vi "GetOneErrorData.vi"(8 "ErrorIn":errorcluster caption="Error In(no Error)", 9 "ErrorCode":i32, 11 "ReferenceIn":refnum<class "ErrorDefinitionSQLite.lvclass"> caption="Reference In") -> (0 "ErrorOut":errorcluster caption="Error Out", 1 "Library":string, 2 "Text":string, 3 "ReferenceOut":refnum<class "ErrorDefinitionSQLite.lvclass"> caption="Reference Out", 4 "Description":string)   [LabVIEW 2018, in "ErrorDefinitionSQLite.lvclass"]
uses:
  ErrorDefinitionSQLite.lvclass
  <vilib>/drjdpowell/SQLite Library/SQL Connection/Execute SQL.vi
  <vilib>/drjdpowell/SQLite Library/SQLite.lvlib
  <vilib>/drjdpowell/SQLite Library/SQL Connection/Connection.lvclass
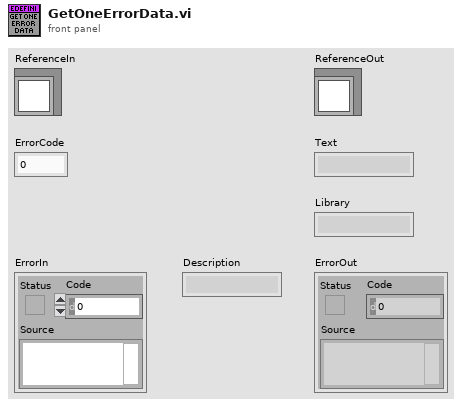
[diagram p1: front panel]
types:
  T1 = typedef "ErrorDefinitionSQLite.lvclass/ObjectAttributes.ctl" = cluster{"Path":path, "SQLiteRef":refnum<class "Connection.lvclass">, "EndOfRange":i32, "DefaultLibrarySize":i32, "StartOfRange":i32}
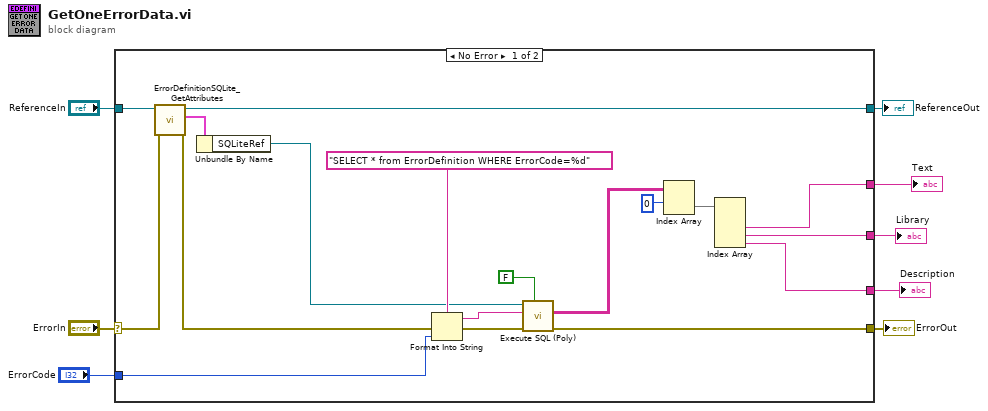
[diagram p0: block diagram]
diagram:
  n1 = case shown="No Error" "ErrorIn" {
    selector: "ErrorIn" -> [w26 w28]
    tunnel: [w9 w28] -> w7
    tunnel: [w24 w27] -> w5
    tunnel: "ReferenceIn" -> [w25 w27]
    tunnel: "ErrorCode" -> [w18 _]
    tunnel: [w14 _] -> w3
    tunnel: [w13 _] -> w2
    tunnel: [w12 _] -> w1
    frame No Error {
      n2 = call "ErrorDefinitionSQLite_GetAttributes.vi"("ErrorIn"=w26, "Reference in"=w25) -> ("ErrorOut"=w10:errorcluster, "Data"=w23:T1, "Reference out"=w24:refnum<class "ErrorDefinitionSQLite.lvclass">)  [unwired: 6 in, 1 out]
      n3 = Unbundle By Name(w23) -> ("SQLiteRef"=w11:refnum<class "Connection.lvclass">)
      n4 = Format Into String(format string="SELECT * from ErrorDefinition WHERE ErrorCode=%d" ("SQL"), error in=w10, w18) -> (resulting string=w20:string, error out=w19:errorcluster)  [unwired: 1 in]
      n5 = call-poly <vilib>:"Execute SQL (Poly).vi"("Use SAVEPOINT"=FALSE, "error in (no error)"=w19, "SQL"=w20, "SQLite Connection in"=w11) -> ("error out"=w9:errorcluster, "Result Set"=w17:string[][])  [unwired: 4 in, 2 out]
      n6 = Index Array(array=w17, index (row)=0 ("disabled index (col)")) -> (element=w15:string[])  [unwired: 1 in]
      n7 = Index Array(array=w15) -> (element #2=w14:string, element #3=w13:string, element #4=w12:string)  [unwired: 4 in, 1 out]
    }
    frame Error {
    }
  }
  "ErrorOut" <- w7
  "ReferenceOut" <- w5
  "Description" <- w1
  "Library" <- w2
  "Text" <- w3
